vi "Find Rows and Columns to draw.vi"(11 "Bounds  Of Picture":T1) -> (1 "Total":u32, 2 "Col":u32, 3 "Rows":u32)   [LabVIEW 2014, in "SmartPalette.lvlib"]
uses:
  SmartPalette.lvlib
  <vilib>/Utility/miscctls.llb/LVBoundsTypeDef.ctl
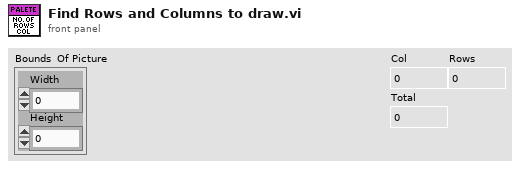
[diagram p1: front panel]
types:
  T1 = typedef "LVBoundsTypeDef.ctl" = cluster{"Width":u32, "Height":u32}
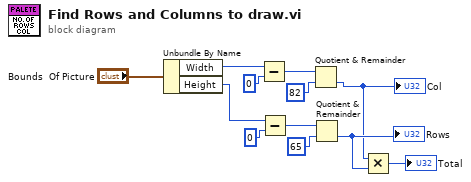
[diagram p0: block diagram]
diagram:
  n1 = Unbundle By Name("Bounds  Of Picture") -> ("Width"=w12:u32, "Height"=w5:u32)
  n2 = Subtract(x=w12, y=u32 0) -> (x-y=w10:u32)
  n3 = Subtract(x=w5, y=u32 0) -> (x-y=w7:u32)
  n4 = Quotient & Remainder(x=w10, y=u32 82) -> (floor(x/y)=w1:u32)  [unwired: 1 out]
  "Col" <- w1
  n5 = Quotient & Remainder(x=w7, y=u32 65) -> (floor(x/y)=w4:u32)  [unwired: 1 out]
  "Rows" <- w4
  n6 = Multiply(x=w1, y=w4) -> (x*y=→"Total":u32)
